vi "Coerce Scale Range to Content.vi"(8 "error in":errorcluster, 11 "Base Graph in":refnum<class "Base Graph.lvclass">) -> (0 "error out":errorcluster, 3 "Base Graph out":refnum<class "Base Graph.lvclass">)   [LabVIEW 2023, in "Base Graph.lvclass"]
uses:
  Base Graph.lvclass
  Base Graph.lvclass/Base Graph.ctl
panel:
  # "PREVENTS AFTER DEZOOMING THE INTENSITY GRAPH IS 1PIXEL TO WIDE"
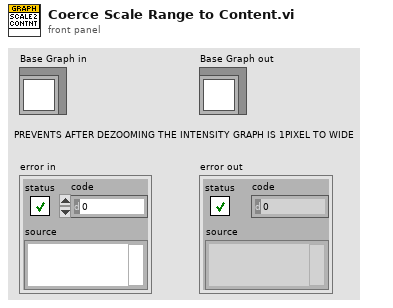
[diagram p1: front panel]
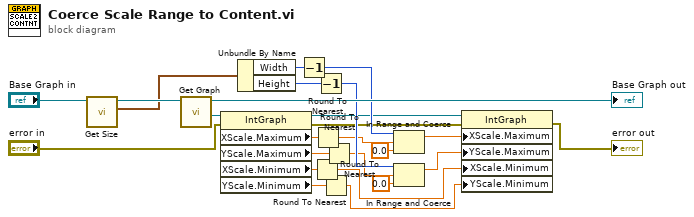
[diagram p0: block diagram]
diagram:
  n1 = call "Get Size.vi"("TG Base Graph in"="Base Graph in") -> ("Sizes"=w20:cluster{"Height":u32, "Width":u32}, "TG Base Graph out"=w22:refnum<class "Base Graph.lvclass">)  [unwired: 9 in]
  n2 = call "Get Graph.vi"("TG Base Graph in"=w22) -> ("Graph"=w21:refnum<vi>, "TG Base Graph out"=→"Base Graph out":refnum<class "Base Graph.lvclass">)  [unwired: 9 in]
  n3 = property class="IntGraph"(reference=w21, error in="error in") -> (reference out=w11:refnum<vi>, error out=w10:errorcluster, "XScale.Maximum"=w19:dbl, "YScale.Maximum"=w15:dbl, "XScale.Minimum"=w7:dbl, "YScale.Minimum"=w6:dbl)
  n4 = Unbundle By Name(w20) -> ("Width"=w18:u32, "Height"=w14:u32)
  n5 = Decrement(x=w18) -> (x-1=w17:u32)
  n6 = Round To Nearest(number=w7) -> (nearest integer value=w3:dbl)
  n7 = Round To Nearest(number=w19) -> (nearest integer value=w5:dbl)
  n8 = Decrement(x=w14) -> (x-1=w13:u32)
  n9 = Round To Nearest(number=w6) -> (nearest integer value=w2:dbl)
  n10 = Round To Nearest(number=w15) -> (nearest integer value=w4:dbl)
  n11 = In Range and Coerce(upper limit=w17, x=w5, lower limit=0.0) -> (coerced(x)=w9:dbl)  [unwired: 1 out]
  n12 = In Range and Coerce(upper limit=w13, x=w4, lower limit=0.0) -> (coerced(x)=w8:dbl)  [unwired: 1 out]
  n13 = property class="IntGraph"(reference=w11, error in=w10, "XScale.Maximum"=w9, "YScale.Maximum"=w8, "XScale.Minimum"=w3, "YScale.Minimum"=w2) -> (error out=→"error out":errorcluster)  [unwired: 1 out]
